vi "Apply Filter_1D.vi"(10 "Filter":string, 11 "Items to Filter":string[](array[string])) -> (3 "Filtered Items":string[](array[string]))   [LabVIEW 2015, in "E2E Tag Exchange editor node.lvclass"]
uses:
  E2E Tag Exchange editor node.lvclass
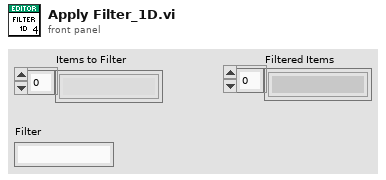
[diagram p1: front panel]
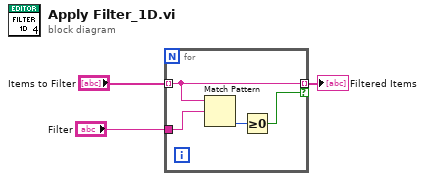
[diagram p0: block diagram]
diagram:
  n1 = for {
    tunnel: "Items to Filter" -> [w6] mode=indexing
    tunnel: "Filter" -> [w7]
    tunnel: [w6] -> w1 mode=indexing if=w4
    n2 = Match Pattern(string=w6, regular expression=w7) -> (offset past match=w5:i32)  [unwired: 1 in, 3 out]
    n3 = Greater Or Equal To 0?(x=w5) -> (x >= 0?=w4:bool)
  }
  "Filtered Items" <- w1
